vi "Practica4.vi"() -> ()   [LabVIEW 2024]
panel:
  out "String de salida constante":string
  out "String de salida":string
  in  "String de entrada":string
  out "Boolean 3":bool
  in  "Boolean 2":bool
  out "Boolean":bool
  out "Area triangulo":dbl
  in  "Altura":dbl
  in  "Base":dbl
  # "Terminal de ENTRADA"
  # "Terminal de SALIDA"
  # "Uso de strings"
  # "Crear cadenas de texto simples"
  # "Controlar instrumentos al enviar comandos de texto al instrumento"
  # "Instruir o advertir al usuario con ventanas de dialogo"
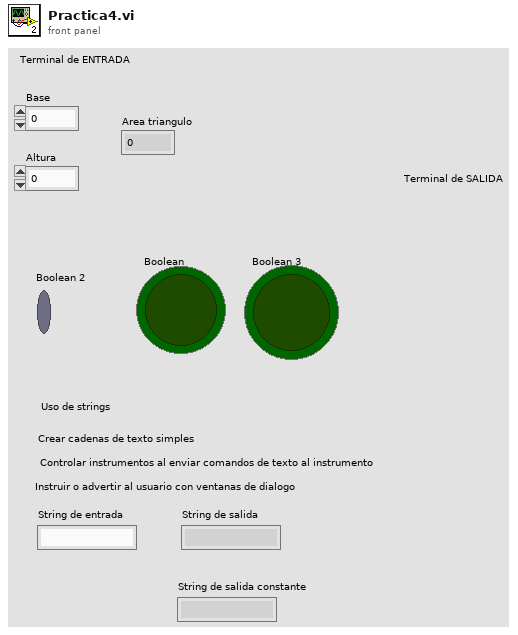
[diagram p1: front panel]
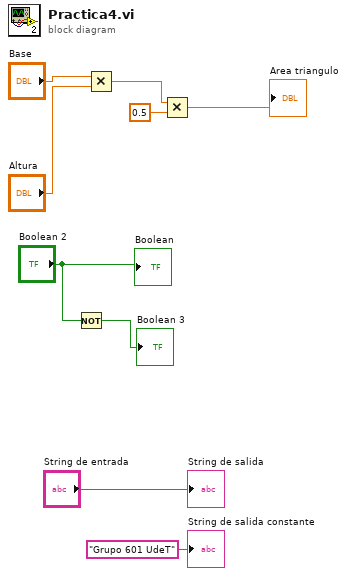
[diagram p0: block diagram]
diagram:
  n1 = Not(x="Boolean 2") -> (.not. x?=→"Boolean 3":bool)
  n2 = Multiply(x="Base", y="Altura") -> (x*y=w7:dbl)
  n3 = Multiply(x=w7, y=0.5) -> (x*y=→"Area triangulo":dbl)
  "Boolean" <- "Boolean 2"
  "String de salida" <- "String de entrada"
  "String de salida constante" <- "Grupo 601 UdeT" ("String de salida constante")
